vi "Alarmas.vi"() -> ()   [LabVIEW 2017]
panel:
  out "Alarmas":T1
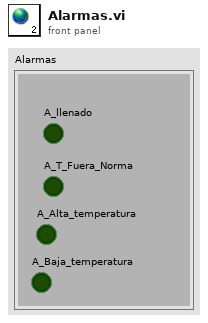
[diagram p1: front panel]
types:
  T1 = cluster{"A_llenado":bool, "A_T_Fuera_Norma":bool, "A_Alta_temperatura":bool, "A_Baja_temperatura ":bool}
diagram:
